vi "Test Complete State.vi"(5 "Queue in":refnum<queue>, 9 "Test Results in":T1, 11 "Error In":errorcluster) -> (10 "Test Results out":T1, 15 "Error Out":errorcluster)   [LabVIEW 2016]
doc: "This VI determines final Pass/Fail of entire test sequence, and updates UI with results."
uses:
  controls/Test Results.ctl
  C:/Program Files (x86)/National Instruments/LabVIEW 2016/examples/Design Patterns/Queued Message Handler/support/QMH Fundamentals - Message Cluster.ctl
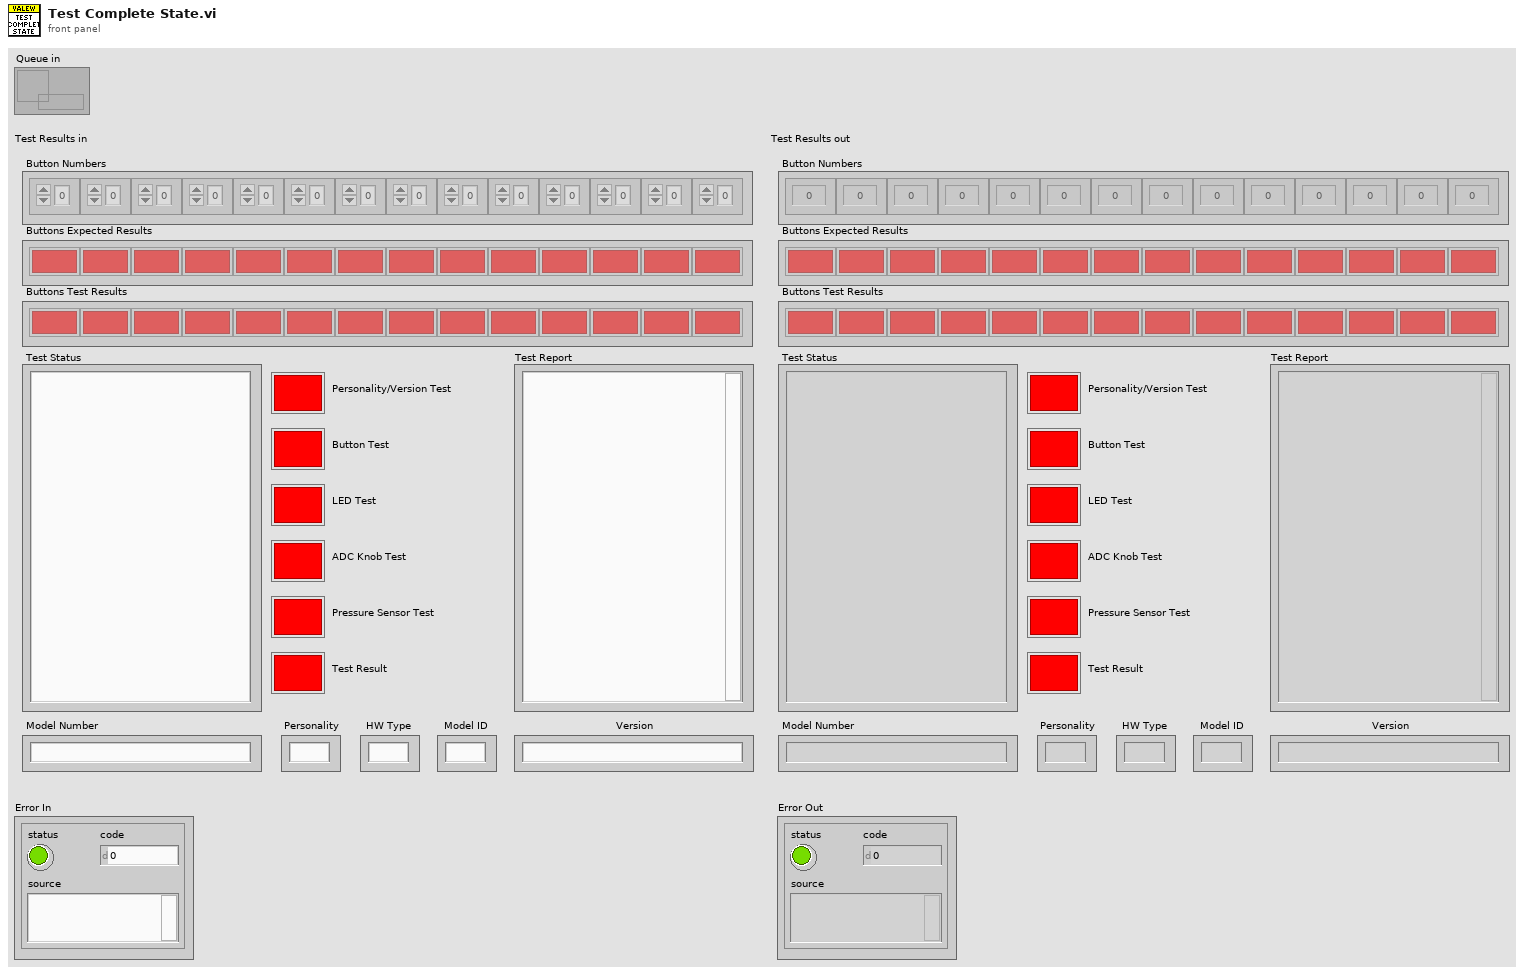
[diagram p1: front panel]
types:
  T1 = typedef "Test Results.ctl" = cluster{"Test Status":string, "Personality/Version Test ":bool, "Test Report":string, "Model Number":string, "Button Numbers":i32[], "Buttons Test Results":bool[], "Buttons Expected Results":bool[], "Model ID":string, "Personality":string, "HW Type":string, "Version":string, "Button Test":bool, "LED Test":bool, "ADC Knob Test":bool, "Pressure Sensor Test":bool, "Test Result":bool}
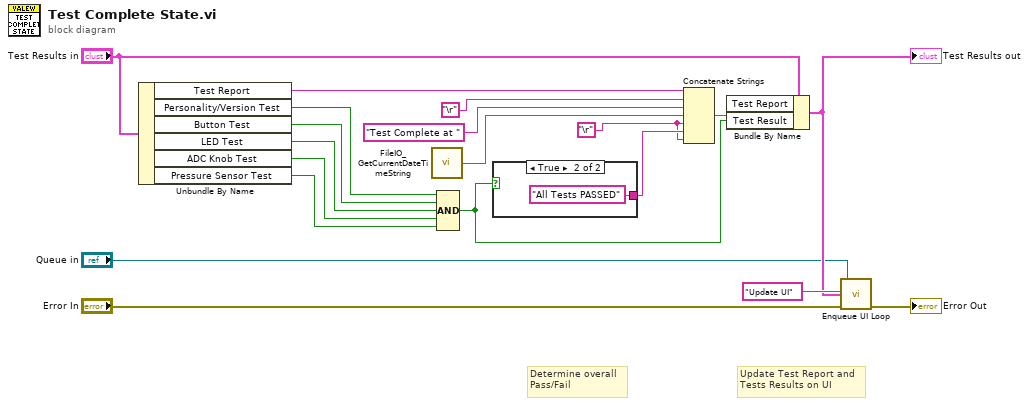
[diagram p0: block diagram]
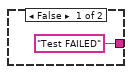
[diagram p2: hidden frame]
diagram:
  w3 = "\r"
  # "Determine overall \nPass/Fail"
  # "Update Test Report and\nTests Results on UI"
  n1 = Unbundle By Name("Test Results in") -> ("Test Report"=w8:string, "Personality/Version Test"=w15:bool, "Button Test"=w16:bool, "LED Test"=w17:bool, "ADC Knob Test"=w2:bool, "Pressure Sensor Test"=w1:bool)
  n2 = call "FileIO_GetCurrentDateTimeString.vi"() -> ("Date/Time String"=w12:string)  [unwired: 14 in, 1 out]
  n3 = Compound Arithmetic op=AND(w15, w16, w17, w2, w1) -> (w18:bool)
  n4 = case shown="True" w18 {
    tunnel: ["Test FAILED" "All Tests PASSED"] -> w19
    frame False {
    }
    frame True {
    }
  }
  n5 = Concatenate Strings(w8, "\r", "Test Complete at " ("Test Status"), w12, w3, w19, w3) -> (w13:string)
  n6 = Bundle By Name(cluster="Test Results in", "Test Report"=w13, "Test Result"=w18) -> (w6:T1)
  "Test Results out" <- w6
  n7 = call "Enqueue UI Loop.vi"("UI Que In"="Queue in", "Message"="Update UI", "Test Results"=w6, "error in (no error)"="Error In") -> ("error out"=→"Error Out":errorcluster)  [unwired: 10 in, 1 out]
